vi "draw.vi"(0 "reference":refnum<class "InterfaceNode.lvclass">, 1 "graphics":refnum<class "Graphics.lvclass">, 5 "error in (no error)":errorcluster) -> (14 "reference out":refnum<class "InterfaceNode.lvclass">, 19 "error out":errorcluster)   [LabVIEW 2012, in "InterfaceNode.lvclass"]
doc: "public void draw(Graphics2D g2, Point2D p, Point2D q)"
uses:
  <resource>/Framework/Providers/Open_GDS/UML/InterfaceNode_class/InterfaceNode.lvclass
  <resource>/Framework/Providers/Open_GDS/UML/Graphics_class/Graphics.lvclass
  <resource>/Framework/Providers/Open_GDS/UML/General/Rectangle/Rectangle Rectangle2D.ctl
  <resource>/Framework/Providers/Open_GDS/UML/MultiLineString_class/MultiLineString.lvclass
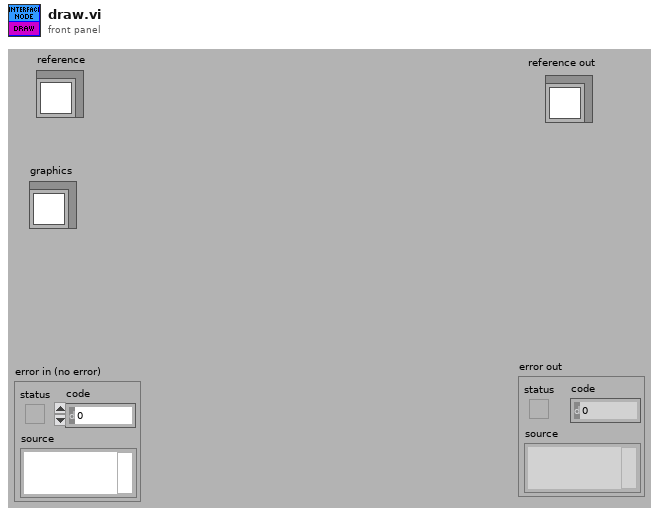
[diagram p1: front panel]
types:
  T1 = typedef "Rectangle Rectangle2D.ctl" = cluster{"x":dbl, "y":dbl, "width":dbl, "height":dbl}
  T2 = typedef "InterfaceNode.lvclass/ObjectAttributes.ctl" = cluster{"Base class":T3, "midHeight":dbl, "botHeight":dbl, "name":refnum<class "MultiLineString.lvclass">, "methods":refnum<class "MultiLineString.lvclass">, "DEFAULT_COMPARTMENT_HEIGHT":i32, "DEFAULT_WIDTH":i32, "DEFAULT_HEIGHT":i32}
  T3 = typedef "RectangularNode.lvclass/ObjectAttributes.ctl" = cluster{"Base class":T4, "bounds":T1}
  T4 = typedef "AbstractNode.lvclass/ObjectAttributes.ctl" = cluster{"parent":refnum<class "AbstractNode.lvclass">, "children":refnum<class "AbstractNode.lvclass">[], "Hidden":bool}
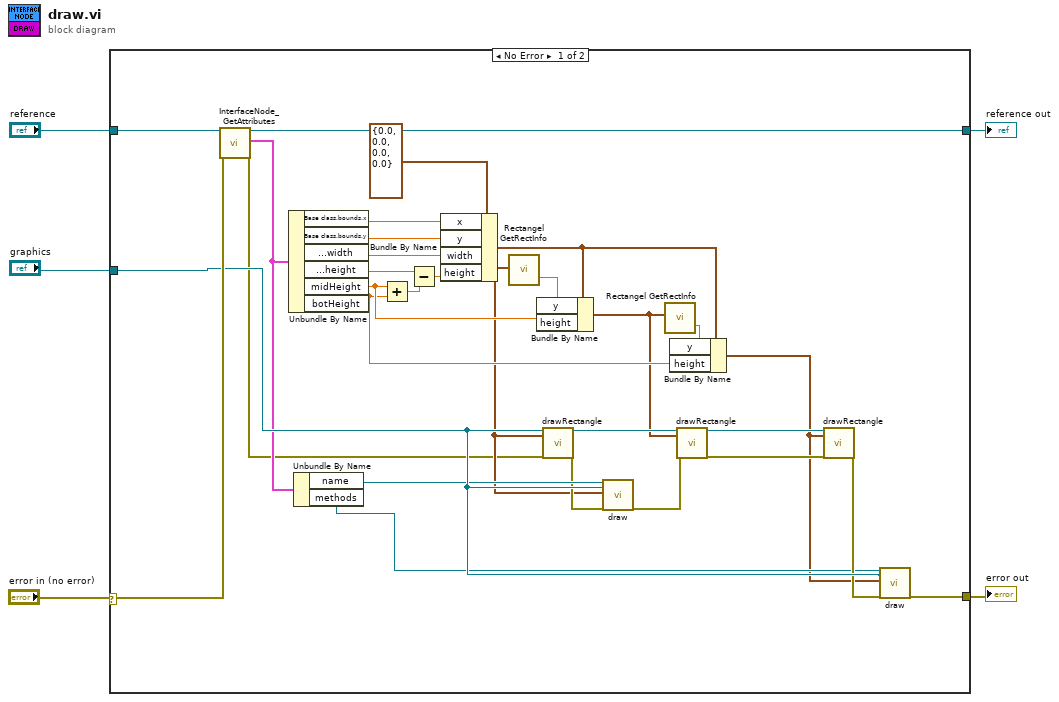
[diagram p0: block diagram]
diagram:
  n1 = case shown="No Error" "error in (no error)" {
    selector: "error in (no error)" -> [w31 w35]
    tunnel: "reference" -> [w34 w36]
    tunnel: [w33 w35] -> w4
    tunnel: [w32 w36] -> w3
    tunnel: "graphics" -> [w30 _]
    frame No Error {
      n2 = call <resource>:"InterfaceNode_GetAttributes.vi"("reference in"=w34, "error in (no error)"=w31) -> ("reference out"=w32:refnum<class "InterfaceNode.lvclass">, "Attributes"=w29:T2, "error out"=w6:errorcluster)  [unwired: 15 out]
      n3 = Unbundle By Name(w29) -> ("Base class.bounds.x"=w27:dbl, "Base class.bounds.y"=w23:dbl, "Base class.bounds.width"=w26:dbl, "Base class.bounds.height"=w25:dbl, "midHeight"=w21:dbl, "botHeight"=w20:dbl)
      n4 = Unbundle By Name(w29) -> ("name"=w17:refnum<class "MultiLineString.lvclass">, "methods"=w12:refnum<class "MultiLineString.lvclass">)
      n5 = Add(x=w21, y=w20) -> (x+y=w22:dbl)
      n6 = Subtract(x=w25, y=w22) -> (x-y=w24:dbl)
      n7 = Bundle By Name(cluster=T1 {"x"=0.0, "y"=0.0, "width"=0.0, "height"=0.0} ("points"), "x"=w27, "y"=w23, "width"=w26, "height"=w24) -> (w9:T1)
      n8 = call <resource>:"Rectangel GetRectInfo.vi"("bounds"=w9) -> ("maxY"=w10:dbl)  [unwired: 1 in, 17 out]
      n9 = Bundle By Name(cluster=w9, "y"=w10, "height"=w21) -> (w8:T1)
      n10 = call <resource>:"drawRectangle.vi"("reference"=w30, "rectangle"=w9, "error in (no error)"=w6) -> ("reference out"=w19:refnum<class "Graphics.lvclass">, "error out"=w16:errorcluster)  [unwired: 4 in, 11 out]
      n11 = call-dynamic "draw.vi"("reference"=w17, "graphics"=w30, "bounds"=w9, "error in (no error)"=w16) -> ("error out"=w15:errorcluster)  [unwired: 14 in, 1 out]
      n12 = call <resource>:"Rectangel GetRectInfo.vi"("bounds"=w8) -> ("maxY"=w7:dbl)  [unwired: 1 in, 17 out]
      n13 = Bundle By Name(cluster=w9, "y"=w7, "height"=w20) -> (w11:T1)
      n14 = call <resource>:"drawRectangle.vi"("reference"=w19, "rectangle"=w8, "error in (no error)"=w15) -> ("reference out"=w18:refnum<class "Graphics.lvclass">, "error out"=w14:errorcluster)  [unwired: 4 in, 11 out]
      n15 = call <resource>:"drawRectangle.vi"("reference"=w18, "rectangle"=w11, "error in (no error)"=w14) -> ("error out"=w13:errorcluster)  [unwired: 4 in, 12 out]
      n16 = call-dynamic "draw.vi"("reference"=w12, "graphics"=w30, "bounds"=w11, "error in (no error)"=w13) -> ("error out"=w33:errorcluster)  [unwired: 14 in, 1 out]
    }
    frame Error {
    }
  }
  "reference out" <- w3
  "error out" <- w4
